vi "Update UI per Reference.vi"(8 "error in (no error)":errorcluster, 11 "Analyze Results Second Momentum in":refnum<class "Analyze Results Second Momentum.lvclass">) -> (0 "error out":errorcluster, 3 "Analyze Results Second Momentum out":refnum<class "Analyze Results Second Momentum.lvclass">)   [LabVIEW 2020, in "Analyze Results Second Momentum.lvclass"]
uses:
  Analyze Results Second Momentum.lvclass
  Analyze Results Second Momentum.lvclass/Analyze Results Second Momentum.ctl
  Results Base/Analyze Results Base.lvclass
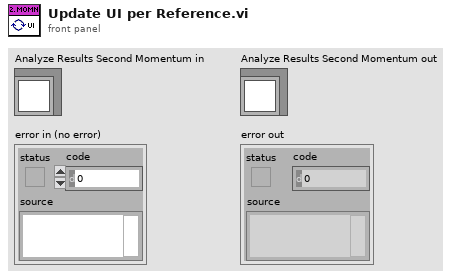
[diagram p1: front panel]
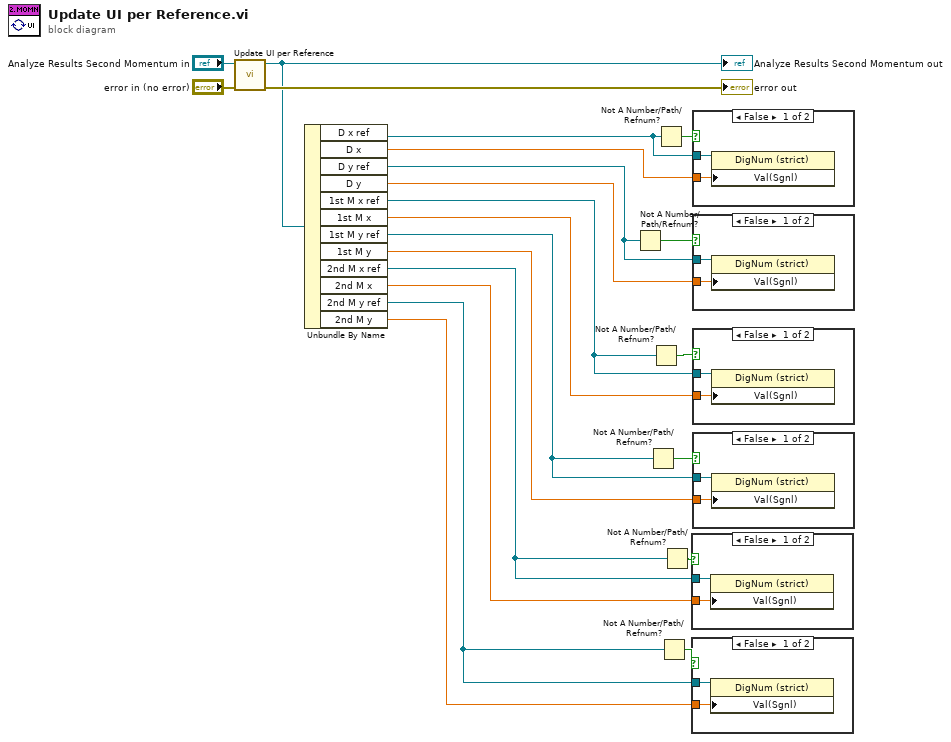
[diagram p0: block diagram]
diagram:
  n1 = call-parent "Update UI per Reference.vi"("error in (no error)"="error in (no error)", "Analyze Results Base in"="Analyze Results Second Momentum in") -> ("error out"=→"error out":errorcluster, "Analyze Results Base out"=w19:refnum<class "Analyze Results Second Momentum.lvclass">)  [unwired: 8 in]
  "Analyze Results Second Momentum out" <- w19
  n2 = Unbundle By Name(w19) -> ("D x ref"=w17:refnum<vi>, "D x"=w16:dbl[unit], "D y ref"=w14:refnum<vi>, "D y"=w13:dbl[unit], "1st M x ref"=w8:refnum<vi>, "1st M x"=w7:dbl[unit], "1st M y ref"=w6:refnum<vi>, "1st M y"=w5:dbl[unit], "2nd M x ref"=w4:refnum<vi>, "2nd M x"=w3:dbl[unit], "2nd M y ref"=w2:refnum<vi>, "2nd M y"=w1:dbl[unit])
  n3 = Not A Number/Path/Refnum?(number/path/refnum=w14) -> (NaN/Path/Refnum?=w15:bool)
  n4 = Not A Number/Path/Refnum?(number/path/refnum=w6) -> (NaN/Path/Refnum?=w12:bool)
  n5 = Not A Number/Path/Refnum?(number/path/refnum=w8) -> (NaN/Path/Refnum?=w11:bool)
  n6 = Not A Number/Path/Refnum?(number/path/refnum=w17) -> (NaN/Path/Refnum?=w18:bool)
  n7 = Not A Number/Path/Refnum?(number/path/refnum=w2) -> (NaN/Path/Refnum?=w9:bool)
  n8 = Not A Number/Path/Refnum?(number/path/refnum=w4) -> (NaN/Path/Refnum?=w10:bool)
  n9 = case shown="False" w10 {
    tunnel: w4 -> [w24 _]
    tunnel: w3 -> [w23 _]
    frame False {
      n10 = property class="DigNum (strict)"(reference=w24, "Val(Sgnl)"=w23) -> ()  [unwired: 1 in, 2 out]
    }
    frame True {
    }
  }
  n11 = case shown="False" w9 {
    tunnel: w2 -> [w26 _]
    tunnel: w1 -> [w25 _]
    frame False {
      n12 = property class="DigNum (strict)"(reference=w26, "Val(Sgnl)"=w25) -> ()  [unwired: 1 in, 2 out]
    }
    frame True {
    }
  }
  n13 = case shown="False" w18 {
    tunnel: w17 -> [w28 _]
    tunnel: w16 -> [w27 _]
    frame False {
      n14 = property class="DigNum (strict)"(reference=w28, "Val(Sgnl)"=w27) -> ()  [unwired: 1 in, 2 out]
    }
    frame True {
    }
  }
  n15 = case shown="False" w15 {
    tunnel: w14 -> [w30 _]
    tunnel: w13 -> [w29 _]
    frame False {
      n16 = property class="DigNum (strict)"(reference=w30, "Val(Sgnl)"=w29) -> ()  [unwired: 1 in, 2 out]
    }
    frame True {
    }
  }
  n17 = case shown="False" w11 {
    tunnel: w8 -> [w32 _]
    tunnel: w7 -> [w31 _]
    frame False {
      n18 = property class="DigNum (strict)"(reference=w32, "Val(Sgnl)"=w31) -> ()  [unwired: 1 in, 2 out]
    }
    frame True {
    }
  }
  n19 = case shown="False" w12 {
    tunnel: w6 -> [w34 _]
    tunnel: w5 -> [w33 _]
    frame False {
      n20 = property class="DigNum (strict)"(reference=w34, "Val(Sgnl)"=w33) -> ()  [unwired: 1 in, 2 out]
    }
    frame True {
    }
  }
